vi "Field Read.vi"(2 "Point #":i32, 3 "Instrument Address":refnum<visa-resource-name>) -> (0 "Stop":bool, 1 "Field":dbl[](array[numeric]) format="%.4e")   [LabVIEW 2021]
doc: "This VI reads almost all types of multimeters and a lot of other IEEE-488 devices single reading mode. The stop boolean is always false. If no reading is obtained a single zero is returned.\nScott Hannahs, NHMFL-FSU, Nov 1993"
panel:
  in  "Type":bool=TRUE
  # "Field [T]"
  # "Current [kA]"
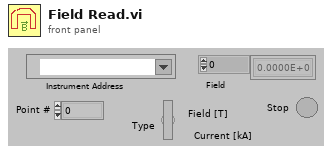
[diagram p1: front panel]
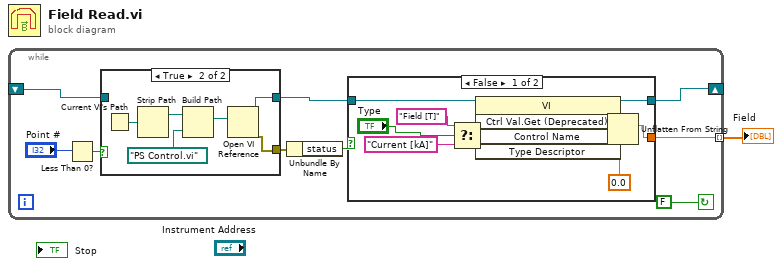
[diagram p0: block diagram]
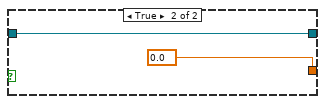
[diagram p2: hidden frame]
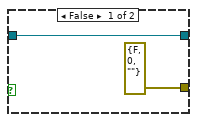
[diagram p3: hidden frame]
diagram:
  n1 = while {
    tunnel: [w5] -> w1 mode=indexing
    shift-left: _ -> [w6]
    shift-right: [w4] -> _
    stop <- FALSE continue-if-true
    n2 = Less Than 0?(x="Point #") -> (x < 0?=w9:bool)
    n3 = case shown="True" w9 {
      tunnel: [w23 w28] -> w7
      tunnel: w6 -> [w23 _]
      tunnel: [errorcluster {"status"=FALSE, "code"=0, "source"=""} ("error out") w29] -> w3
      frame False {
      }
      frame True {
        n4 = Current VI's Path() -> (path=w25:path)
        n5 = Strip Path(path=w25) -> (stripped path=w27:path)  [unwired: 1 out]
        n6 = Build Path(base path=w27, name or relative path=path "PS Control.vi") -> (appended path=w24:path)
        n7 = Open VI Reference(vi path=w24) -> (vi reference=w28:refnum<vi>, error out=w29:errorcluster)  [unwired: 5 in]
      }
    }
    n8 = Unbundle By Name(w3) -> ("status"=w8:bool)
    n9 = case shown="False" w8 {
      tunnel: w7 -> [w19 w20]
      tunnel: [w16 0.0] -> w5
      tunnel: [w15 w20] -> w4
      frame False {
        n10 = Select(t="Field [T]" ("Control Name"), s="Type", f="Current [kA]") -> (s? t:f=w14:string)
        n11 = invoke class="VI" method="Ctrl Val.Get (Deprecated)"(reference=w19, "Control Name"=w14) -> (reference out=w15:refnum<vi>, "Get Control Value"=w18:string)  [unwired: 3 in, 3 out]
        n12 = Unflatten From String(type=0.0, binary string=w18) -> (value=w16:dbl)  [unwired: 3 in, 2 out]
      }
      frame True {
      }
    }
  }
  "Field" <- w1
